vi "Destroy.vi"(8 "error in (no error)":errorcluster, 11 "CIFTag in":refnum<class "CIF_CIPC_Chn.lvclass">) -> (0 "error out":errorcluster, 3 "CIFTag out":refnum<class "CIF_CIPC_Chn.lvclass">)   [LabVIEW 2021, in "CIF_CIPC_Chn.lvclass"]
uses:
  CIF_CIPC_Chn.lvclass
  D:/dev/Packages/CIF_Channels_Core/src/CIFChannels/CIFChannels.lvclass
  Typedef/Buffer Configuration Data.ctl
  <vilib>/CIF Foundation/CIF CIPC/TypeDefs/Backpressure References.ctl
  CIFChannels/CIFChannels.lvclass/CIFChannels.ctl
  CIF_CIPC_Chn.lvclass/CIF_CIPC_Chn.ctl
  CIFChannels/Accessors/Read Direction.vi
  CIFChannels/Accessors/Read FIFO Backpressure.vi
  Accessors/Read Buffer Configuration.vi
  Accessors/Read CIPC Channel.vi
  Accessors/Write Buffer Configuration.vi
  Accessors/Write CIPC Channel.vi
  <vilib>/CIF Foundation/CIF CIPC/CIF_NI_CIPC.lvlib
  CIFChannels/Typedef/Channel State.ctl
  CIFChannels/CIFChannels.lvclass
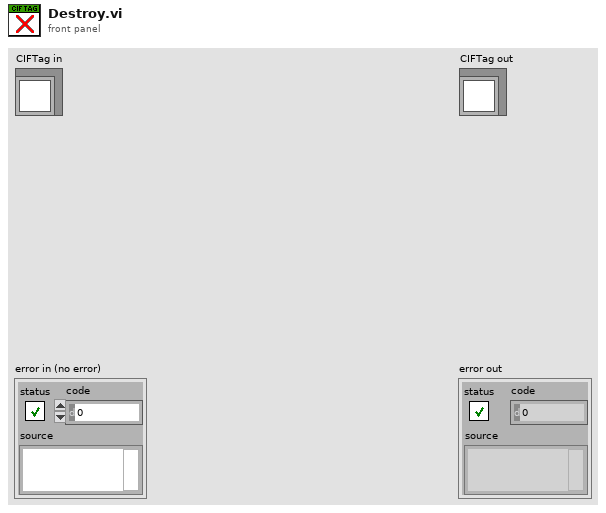
[diagram p1: front panel]
types:
  T1 = typedef "CIFChannels.lvclass/Channel State.ctl" = enum16{"Creating", "Disconnected", "Connecting", "Connected", "Destroyed"}
  T2 = typedef "CIF_CIPC_Chn.lvclass/Buffer Configuration Data.ctl" = cluster{"Total Size":u32, "Read Size":u32, "Read Offset":u32, "CIPC BP References":T3, "Override CIPC Name":string, "Encoder Data":string}
  T3 = typedef "CIF_NI_CIPC.lvlib/Backpressure References.ctl" = cluster{"CIPC Reference":u64, "CIPC BP Reference":u64}
  T4 = typedef "CIFChannels.lvclass/Direction.ctl" = enum16{"Publisher", "Subscriber"}
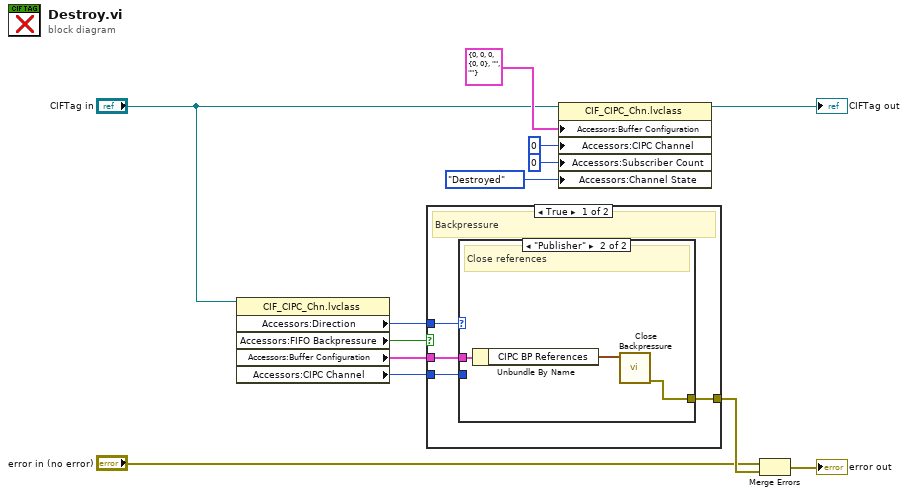
[diagram p0: block diagram]
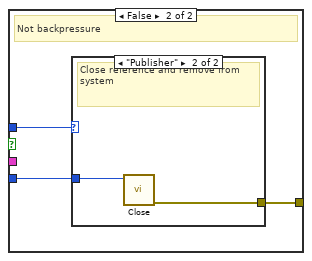
[diagram p3: hidden frame]
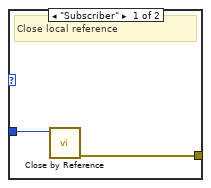
[diagram p4: hidden frame]
diagram:
  n1 = property class="CIF_CIPC_Chn.lvclass"(reference="CIFTag in") -> ("Accessors:Direction"=w13:T4, "Accessors:FIFO Backpressure"=w11:bool, "Accessors:Buffer Configuration"=w10:T2, "Accessors:CIPC Channel"=w12:u64)  [unwired: 1 in, 2 out]
  n2 = case shown="True" w11 {
    tunnel: w13 -> [w17 w23]
    tunnel: w12 -> [w16 w22]
    tunnel: [w14 w21] -> w9
    tunnel: w10 -> [w15 _]
    frame True {
      # "Backpressure"
      n3 = case shown="\"Publisher\"" w17 {
        tunnel: w16 -> [_ _]
        tunnel: w15 -> [_ w20]
        tunnel: [_ w18] -> w14
        frame "Subscriber" {
          # "Backpressure references owned and closed by publisher"
        }
        frame "Publisher" {
          # "Close references"
          n4 = Unbundle By Name(w20) -> ("CIPC BP References"=w19:T3)
          n5 = call <vilib>:"Close Backpressure.vi"("CIPC BP References in"=w19) -> ("error out"=w18:errorcluster)  [unwired: 10 in]
        }
      }
    }
    frame False {
      # "Not backpressure"
      n6 = case shown="\"Publisher\"" w23 {
        tunnel: w22 -> [w25 w27]
        tunnel: [w24 w26] -> w21
        frame "Subscriber" {
          # "Close local reference"
          n7 = call <vilib>:"Close by Reference.vi"("CIPC Reference"=w25) -> ("error out"=w24:errorcluster)  [unwired: 10 in]
        }
        frame "Publisher" {
          # "Close reference and remove from system"
          n8 = call <vilib>:"Close.vi"("CIPC Reference"=w27) -> ("error out"=w26:errorcluster)  [unwired: 10 in]
        }
      }
    }
  }
  n9 = property class="CIF_CIPC_Chn.lvclass"(reference="CIFTag in", "Accessors:Buffer Configuration"=T2 {"Total Size"=0, "Read Size"=0, "Read Offset"=0, "CIPC BP References"={"CIPC Reference"=0, "CIPC BP Reference"=0}, "Override CIPC Name"="", "Encoder Data"=""} ("Buffer Configuration"), "Accessors:CIPC Channel"=u64 0 ("CIPC Channel"), "Accessors:Subscriber Count"=u32 0 ("Subscriber Count"), "Accessors:Channel State"=Channel_State."Destroyed" ("Channel State")) -> (reference out=→"CIFTag out":refnum<class "CIF_CIPC_Chn.lvclass">)  [unwired: 1 in, 1 out]
  n10 = Merge Errors("error in (no error)", w9) -> (→"error out":errorcluster)
